vi "Create New Limits File.vi"(8 "error in (no error)":errorcluster, 10 "Test Modes":string[](array[string]), 11 "Limits File Path":path) -> (0 "error out":errorcluster)   [LabVIEW 2018, in "Test Number and Bin Generator.lvlib" / "Test Number and Bin Generator.lvclass"]
uses:
  Test Number and Bin Generator.lvclass
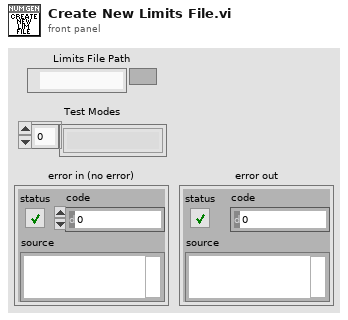
[diagram p1: front panel]
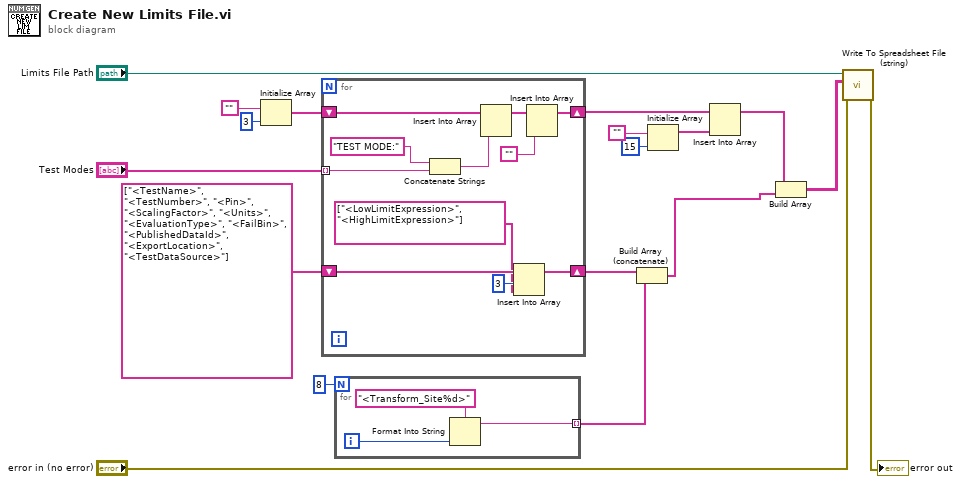
[diagram p0: block diagram]
diagram:
  n1 = Initialize Array("", 3 ("dimension size")) -> (w10:string[])
  n2 = for {
    shift-right: [w27] -> w14
    shift-left: w10 -> [w29]
    tunnel: "Test Modes" -> [w26] mode=indexing
    shift-right: [w19] -> w3
    shift-left: string[] ["<TestName>", "<TestNumber>", "<Pin>", "<ScalingFactor>", "<Units>", "<EvaluationType>", "<FailBin>", "<PublishedDataId>", "<ExportLocation>", "<TestDataSource>"] -> [w22]
    n3 = Concatenate Strings("TEST MODE:" ("string"), w26) -> (w24:string)
    n4 = Insert Into Array(array=w29, new element=w24) -> (w28:string[])  [unwired: 1 in]
    n5 = Insert Into Array(array=w22, index=3, new element=string[] ["<LowLimitExpression>", "<HighLimitExpression>"]) -> (w19:string[])
    n6 = Insert Into Array(array=w28, new element="") -> (w27:string[])  [unwired: 1 in]
  }
  n7 = for {
    N: 8 -> [_]
    tunnel: [w30] -> w2 mode=indexing
    i -> [w32]
    n8 = Format Into String(format string="<Transform_Site%d>", w32) -> (resulting string=w30:string)  [unwired: 2 in, 1 out]
  }
  n9 = Build Array (concatenate)(w3, w2) -> (w1:string[])
  n10 = Initialize Array("", 15 ("dimension size")) -> (w15:string[])
  n11 = Insert Into Array(array=w14, new element=w15) -> (w17:string[])  [unwired: 1 in]
  n12 = Build Array(w17, w1) -> (w18:string[][])
  n13 = call "Write To Spreadsheet File (string).vi"("file path (dialog if empty)"="Limits File Path", "2D data"=w18, "error in"="error in (no error)") -> ("error out"=→"error out":errorcluster)  [unwired: 6 in, 1 out]
